vi "Process.vi"(8 "error in":errorcluster, 11 "Measurement.WavelengthSweeping":refnum<class "Measurement.WavelengthSweeping.lvclass">) -> (0 "error out":errorcluster, 3 "Measurement.WavelengthSweeping out":refnum<class "Measurement.WavelengthSweeping.lvclass">)   [LabVIEW 2017, in "Measurement.WavelengthSweeping.lvclass"]
doc: "---------------------------------------------------------------\nJKI State Machine Objects™\nhttp://jki.net/state-machine-objects/\nCopyright (C) 2005-2015, JKI <info@jki.net>\nALL RIGHTS RESERVEDJKI State Machine Objects (SMO) 1.0.0.5\nJKI - JKI\nCopyright (c) 2016, JKI"
uses:
  Measurement.WavelengthSweeping.lvclass
  D:/Program Files (x86)/National Instruments/LabVIEW 2017/vi.lib/JKI/JKI SMO/SMO/SMO.lvclass
  D:/upwork/Laser Measurement Tool/Laser/project/Subsystems/Measurement/Measurement.lvclass
  <vilib>/JKI/JKI SMO/SMO/Typedefs/Parent Call--Enum.ctl
  Measurement/Typedefs/Measurement.State--Enum.ctl
  OPA/Typedefs/PrivateEvents--OPA.SetShutterState.ctl
  Typedefs/Measurement.WavelengthSweeping.State--Enum.ctl
  Typedefs/Measurement.WavelengthSweeping.Measured--Data.ctl
  Measurement/Typedefs/PublicEvents--Measurement.Finished.ctl
  Measurement/Typedefs/PublicEvents--Measurement.Initialized.ctl
  <vilib>/Analysis/baseanly.llb/Mean (DBL).vi
  SMU/SMU.lvclass
  D:/upwork/Laser Measurement Tool/Laser/project/Subsystems/MeasuringDevice/MeasuringDevice.lvclass
  LIA/LIA.lvclass
  OPM/OPM.lvclass
  Measurement/Measurement.lvclass
  <vilib>/JKI/JKI SMO/SMO/SMO.lvclass
  OPA/OPA.lvclass
  MeasuringDevice/MeasuringDevice.lvclass
  <vilib>/Analysis/NI_AALBase.lvlib
panel:
  # "Measurement.WavelengthSweeping\nProcess.vi"
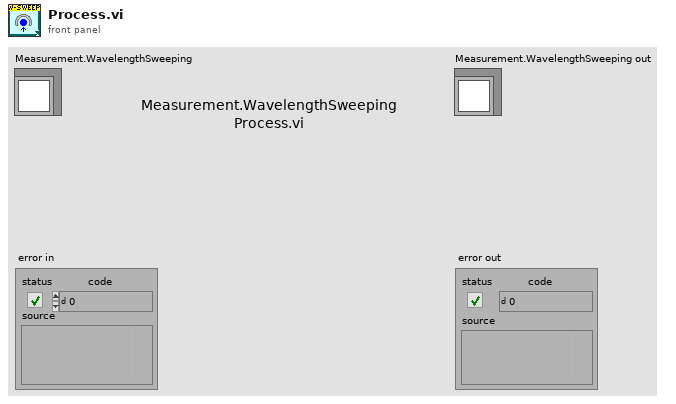
[diagram p1: front panel]
types:
  T1 = typedef "SMO.lvclass/Parent Call--Enum.ctl" = enum16{"Allows parent to run", "Does not request parent to run"}
  T2 = typedef "Measurement.lvclass/Measurement.State--Enum.ctl" = enum16{"Uninitialized", "Initialized", "Started", "Paused", "Stopped"}
  T3 = typedef "OPA.lvclass/PrivateEvents--OPA.SetShutterState.ctl" = bool
  T4 = typedef "Measurement.WavelengthSweeping.lvclass/Measurement.WavelengthSweeping.State--Enum.ctl" = enum16{"Stoppped", "Wait for Wavelength set", "Wait for Integration time", "Wait for Measurements", "Wait for Delay time"}
  T5 = enum32{"invalid app kind", "Development System", "Run Time System", "Student Edition", "Embedded LabVIEW", "Evaluation", "Custom"}
  T6 = enum32{"Invalid", "Standard", "Closed", "Hidden", "Minimized", "Maximized"}
  T7 = typedef "Measurement.lvclass/PublicEvents--Measurement.Finished.ctl" = bool
  T8 = typedef "Measurement.lvclass/PublicEvents--Measurement.Initialized.ctl" = bool
  T9 = typedef "Measurement.WavelengthSweeping.lvclass/Dependencies--Cluster.ctl" = cluster{"SMU":refnum<class "SMU.lvclass">, "LIA":refnum<class "LIA.lvclass">, "OPM":refnum<class "OPM.lvclass">, "OPA":refnum<class "OPA.lvclass">}
  T10 = typedef "Measurement.WavelengthSweeping.lvclass/Configuration--Cluster.ctl" = cluster{"Measurement.Type":T11, "Hardware":T12, "Measurement":T21}
  T11 = typedef "Measurement.lvclass/Measurement.Type--Enum.ctl" = enum16{"Free", "I/V Curve", "Wavelength sweeping", "Photocurrent mapping"}
  T12 = typedef "Measurement.WavelengthSweeping.lvclass/Configuration.Hardware--Cluster.ctl" = cluster{"SMU":T13, "LIA":T15, "OPM":T17, "OPA":T19}
  T13 = typedef "Measurement.lvclass/Configuration.SMU--Cluster.ctl" = cluster{"Enable":bool, "SMU Model":string, "Configuration":T14}
  T14 = typedef "SMU.lvclass/Configuration--Cluster.ctl" = cluster{"VISA Resource":string, "Channel":string}
  T15 = typedef "Measurement.lvclass/Configuration.LIA--Cluster.ctl" = cluster{"Enable":bool, "LIA Model":string, "Configuration":T16}
  T16 = typedef "LIA.lvclass/Configuration--Cluster.ctl" = cluster{"VISA Resource":string}
  T17 = typedef "Measurement.lvclass/Configuration.OPM--Cluster.ctl" = cluster{"Enable":bool, "OPM Model":string, "Configuration":T18}
  T18 = typedef "OPM.lvclass/Configuration--Cluster.ctl" = cluster{"VISA Resource":string}
  T19 = typedef "Measurement.lvclass/Configuration.OPA--Cluster.ctl" = cluster{"Enable":bool, "OPA Model":string, "Configuration":T20}
  T20 = typedef "OPA.lvclass/Configuration--Cluster.ctl" = cluster{"Serial Number":string}
  T21 = typedef "Measurement.WavelengthSweeping.lvclass/Configuration.Measurement--Cluster.ctl" = cluster{"SMU Voltage, V":dbl, "OPA Start wavelength, nm":dbl, "OPA Stop wavelength, nm":dbl, "OPA Scan resolution, nm":dbl, "OPA Number or points":u16, "Integration time, sec":dbl, "Delay time, ms":u16, "Accumulation":u16}
  T22 = cluster{"Core":cluster{"Current VI Reference":refnum<vi>, "Close Panel on Exit?":bool, "error":errorcluster}, "Self Reference":refnum<class "Measurement.WavelengthSweeping.lvclass">, "Dependencies":T9, "Configuration":T10, "Initialized":bool, "Meas State":T2, "W-Sweep State":T4, "Flags":cluster{"SMU Completed":bool, "LIA Completed":bool, "OPM Completed":bool, "OPA Wavelength":bool, "OPA Shutter State":bool}, "Next Step":string, "Wavelength, nm":dbl, "Start Time":timestamp, "SMU Measurement":dbl, "LIA Measurement":dbl, "OPM Measurement":dbl}
  T23 = cluster{"SMU Completed":bool, "LIA Completed":bool, "OPM Completed":bool, "OPA Wavelength":bool, "OPA Shutter State":bool}
  T24 = cluster{"Current VI Reference":refnum<vi>, "Close Panel on Exit?":bool, "error":errorcluster}
  T25 = typedef "Measurement.WavelengthSweeping.lvclass/Measurement.WavelengthSweeping.Measured--Data.ctl" = cluster{"Wavelength, nm":dbl, "Power, W":dbl, "Current, A":dbl, "Magnitude":dbl}
  T26 = typedef "SMO.lvclass/Protected Events.ctl" = cluster{"StopProcesses":refnum<user-event>, "AbortProcesses":refnum<user-event>, "Config Changed":refnum<user-event>, "Dependency":refnum<user-event>}
  T27 = cluster{"Event Registration Refnum":refnum<event-registration>, "Measurement Protected Events":refnum<event-registration>, "SMU Public Events":refnum<event-registration>, "LIA Public Events":refnum<event-registration>, "OPM Public Events":refnum<event-registration>, "OPA Public Events":refnum<event-registration>}
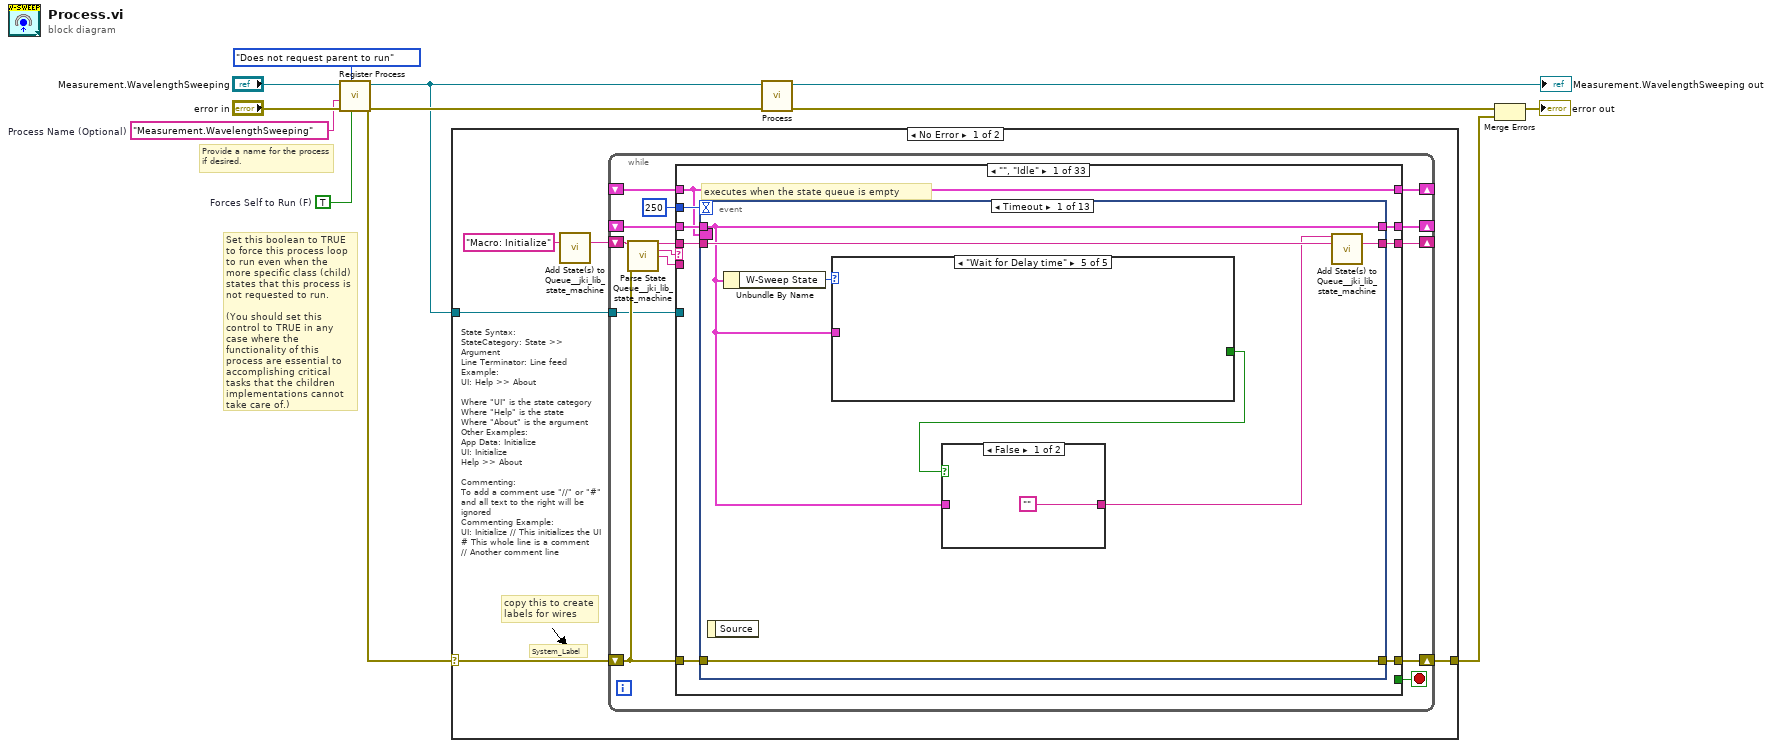
[diagram p0: block diagram]
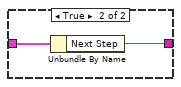
[diagram p2: hidden frame]
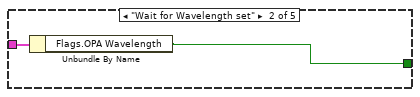
[diagram p4: hidden frame]
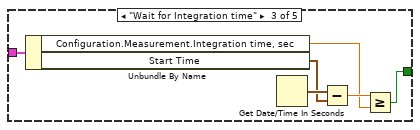
[diagram p5: hidden frame]
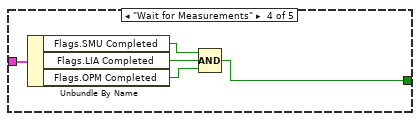
[diagram p6: hidden frame]
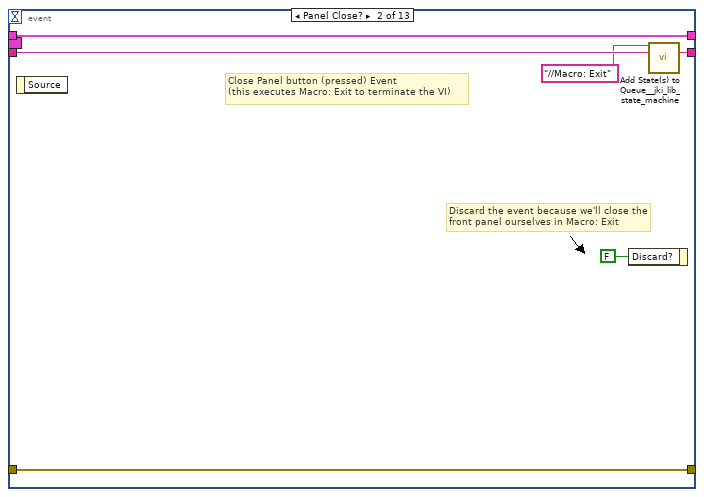
[diagram p7: hidden frame]
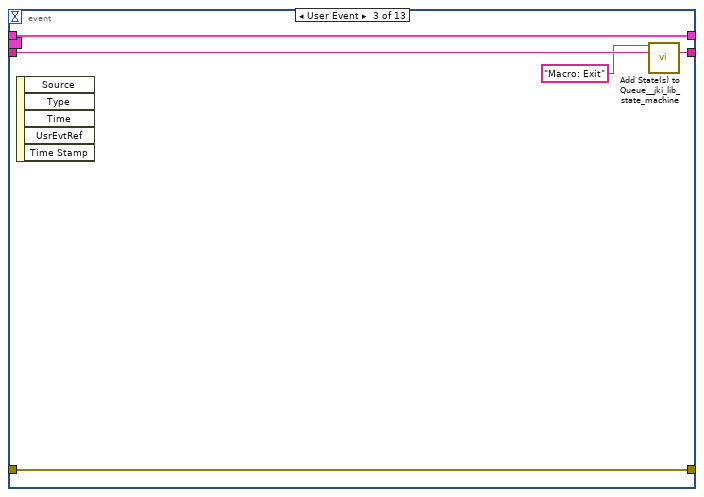
[diagram p8: hidden frame]
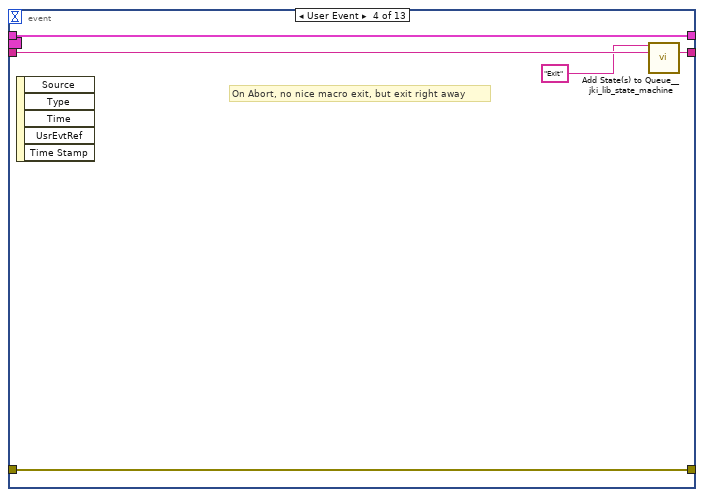
[diagram p9: hidden frame]
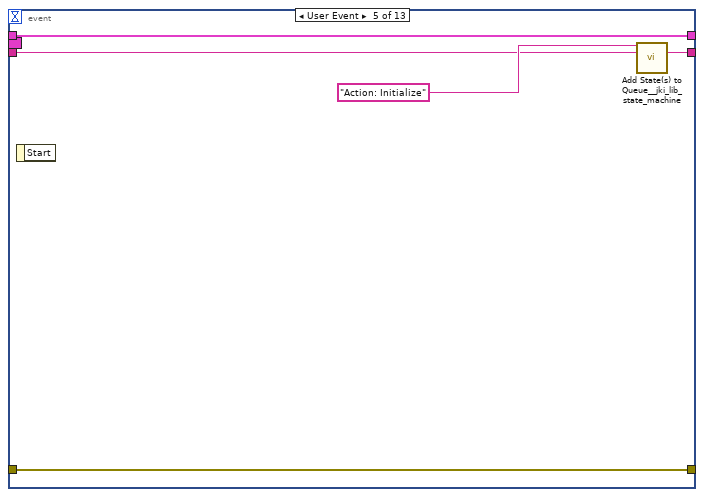
[diagram p10: hidden frame]
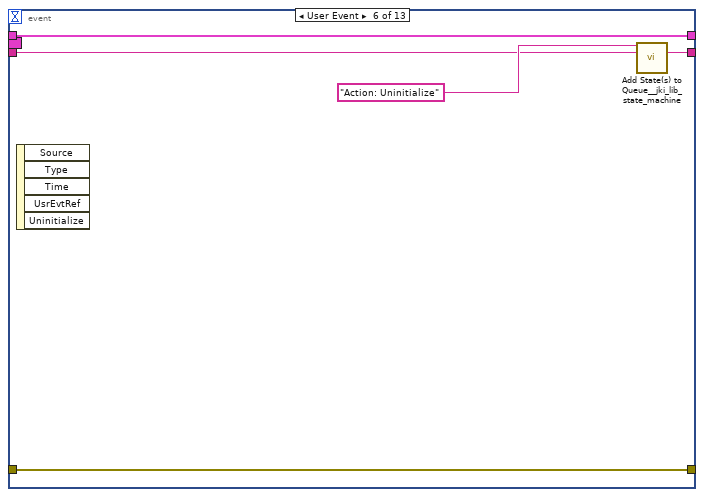
[diagram p11: hidden frame]
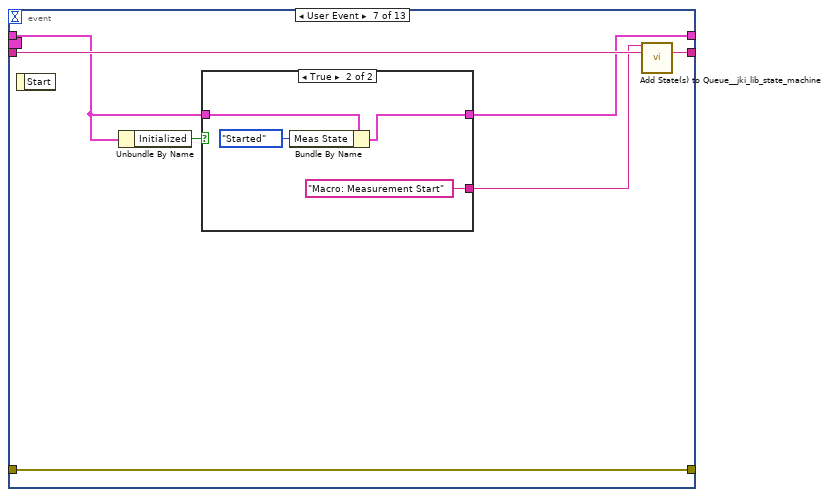
[diagram p12: hidden frame]
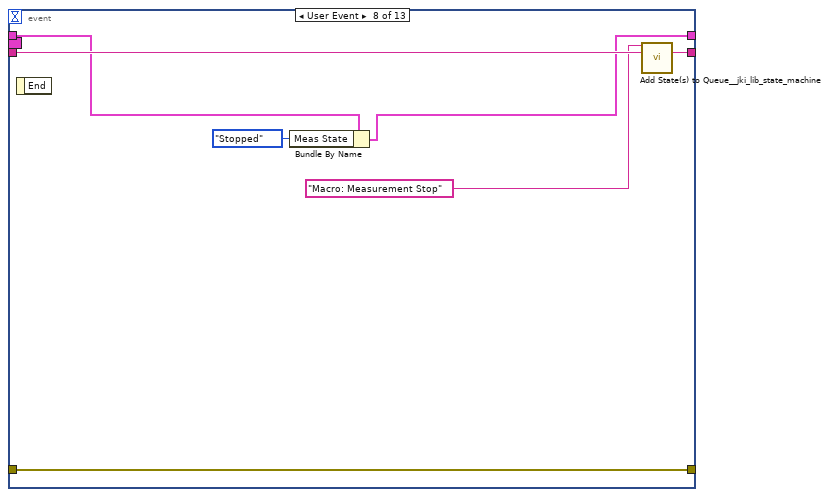
[diagram p14: hidden frame]
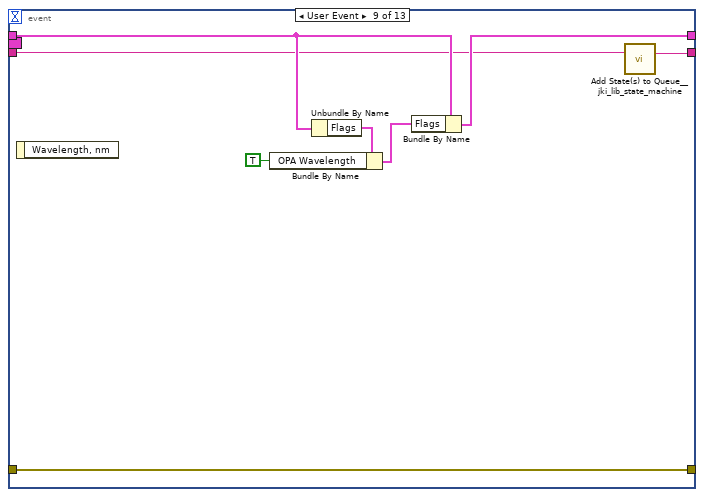
[diagram p15: hidden frame]
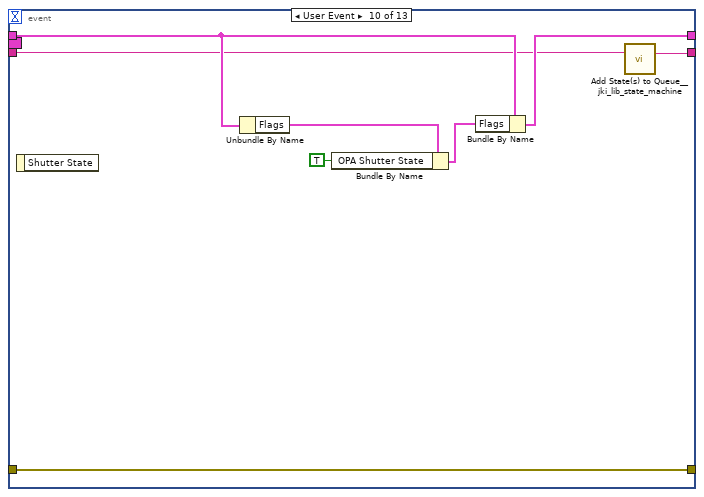
[diagram p16: hidden frame]
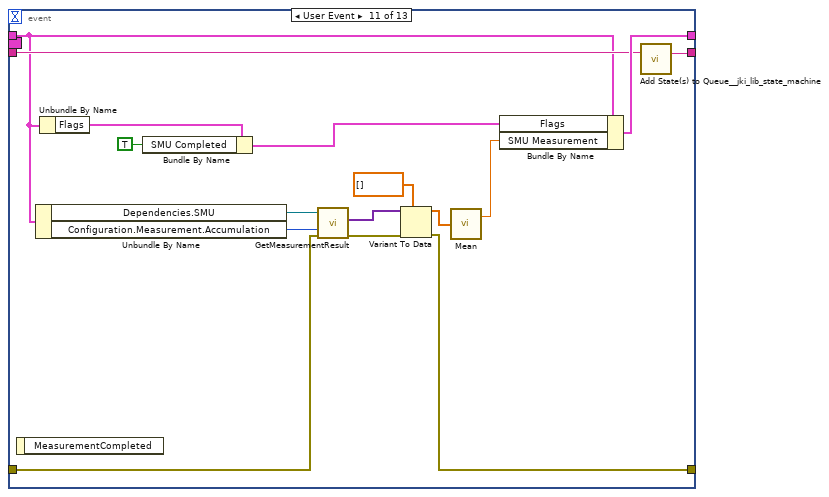
[diagram p17: hidden frame]
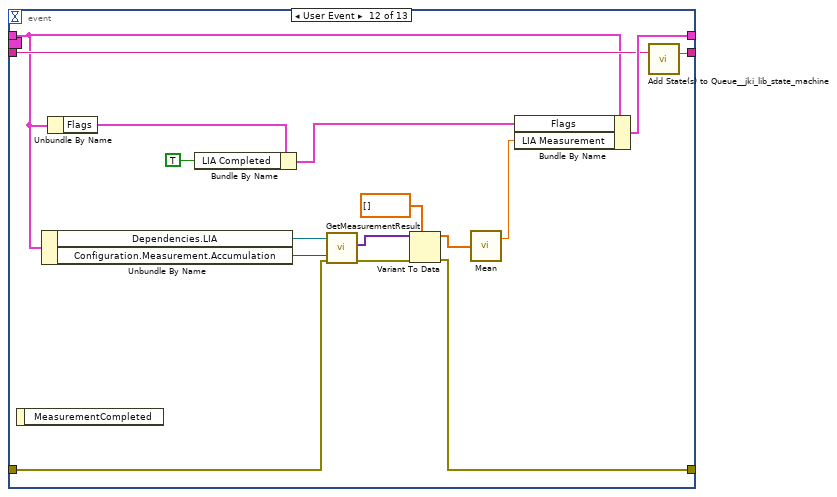
[diagram p18: hidden frame]
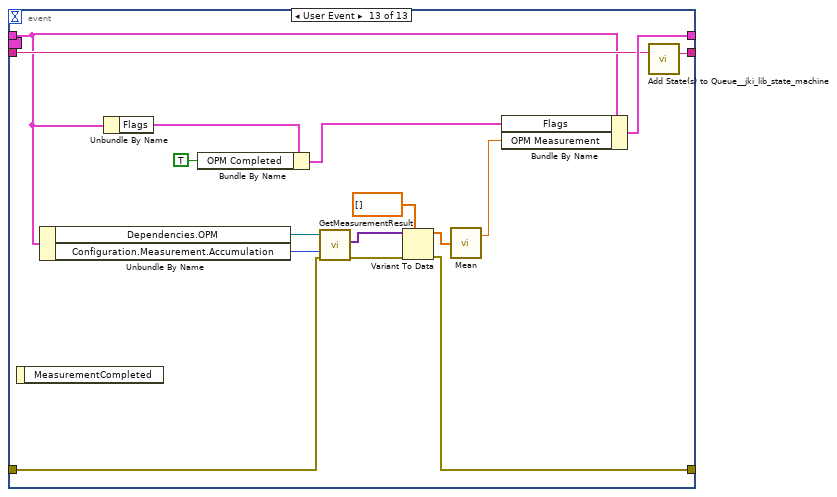
[diagram p19: hidden frame]
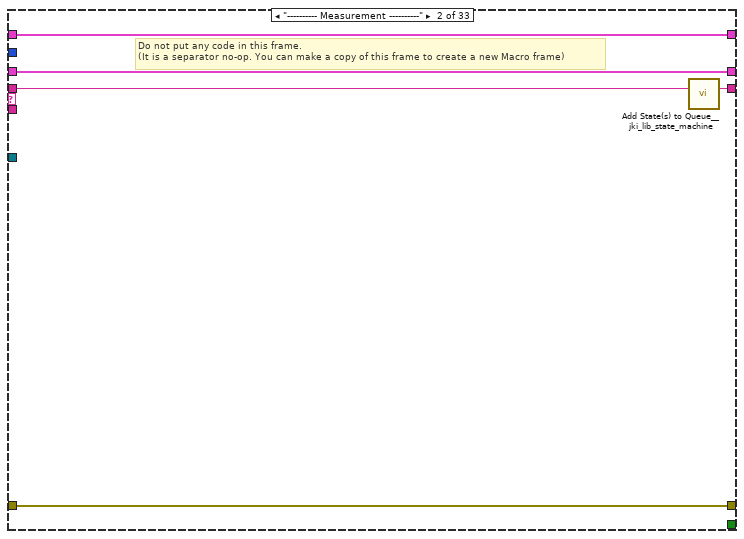
[diagram p20: hidden frame]
diagram:
  w2 = TRUE  # Forces Self to Run (F)
  w1 = "Measurement.WavelengthSweeping"  # Process Name (Optional)
  # "Provide a name for the process\nif desired."
  # "Set this boolean to TRUE to force this process loop to run even when the more specific class (child) states that this process is not requested to run.\n\n(You should set this control to TRUE in any case where the functionality of this process are essential to accomplishing critical tasks that the children implementations cannot take care of.)"
  n1 = call <vilib>:"Register Process.vi"("Forces Self to Run (F)"=w2, "Parent Call"=Parent_Call--Enum."Does not request parent to run", "error in (no error)"="error in", "Process Name (optional)"=w1, "SMO"="Measurement.WavelengthSweeping") -> ("error out"=w8:errorcluster, "SMO out"=w7:refnum<class "Measurement.WavelengthSweeping.lvclass">)  [unwired: 5 in]
  n2 = case shown="No Error" w8 {
    selector: w8 -> [w13 w662]
    tunnel: w7 -> [w14 _]
    tunnel: [w12 w662] -> w4
    frame No Error {
      # "State Syntax:\nStateCategory: State >> Argument\nLine Terminator: Line feed\nExample:\nUI: Help >> About\n\nWhere \"UI\" is the state category\nWhere \"Help\" is the state\nWhere \"About\" is the argument\nOther Examples:\nApp Data: Initialize\nUI: Initialize\nHelp >> About\n\nCommenting:\nTo add a comment use \"//\" or \"#\" and all text to the right will be ignored\nCommenting Example:\nUI: Initialize // This initializes the UI\n# This whole line is a comment\n// Another comment line"
      # "copy this to create labels for wires"
      # "System_Label"
      n3 = call <vilib>:"Add State(s) to Queue__jki_lib_state_machine.vi"("State(s) in (\"\")"="Macro: Initialize") -> ("States Out"=w16:string)  [unwired: 14 in]
      n4 = while {
        shift-right: [w23] -> _
        shift-left: _ -> [w22]
        shift-right: [w26] -> w12
        shift-left: w13 -> [w20]
        shift-right: [w25] -> _
        shift-left: w16 -> [w27]
        tunnel: w14 -> [w19]
        shift-right: [w18] -> _
        shift-left: _ -> [w17]
        stop <- w24 stop-if-true
        n5 = call <vilib>:"Parse State Queue__jki_lib_state_machine.vi"("State Queue"=w27, "Error In (no error)"=w20) -> ("Remaining States"=w29:string, "Current State"=w30:string, "Arguments"=w28:string)  [unwired: 11 in]
        n6 = case shown="\"\", \"Idle\"" w30 {
          selector: w30 -> [_ _ w176 w207 w258 w282 _ _ w363 _ _ _ _ _ _ _ _ _ _ _ _ _ _ _ _ _ _ _ _ _ _ _ _]
          tunnel: w29 -> [w38 w175 w183 w215 w264 w291 w348 w361 w367 w386 w401 w407 w412 w437 w444 w449 w454 w461 w477 w518 w523 w532 w546 w558 w571 w576 w587 w592 w617 w623 w628 w641 w661]
          tunnel: w28 -> [_ _ w181 w213 w261 w288 _ _ _ _ _ _ _ _ _ _ _ w455 w471 _ _ _ _ _ _ _ _ _ _ _ _ _ _]
          tunnel: w22 -> [w36 w172 w179 w211 w260 w284 w340 w358 w365 w377 w391 w403 w409 _ w439 w446 w452 w459 w473 w515 w520 w528 w537 w553 w563 w573 w584 w589 w596 w621 w626 w633 w652]
          tunnel: [w35 w173 w177 w209 w256 w285 w346 w359 w369 w383 w393 w402 w410 w425 w440 w447 w451 w456 w474 w507 w521 w530 w544 w556 w560 w574 w578 w590 w612 w619 w624 w629 w654] -> w26
          tunnel: w20 -> [w34 w173 w178 w210 w257 w286 w346 w359 w368 w383 w388 _ w410 w434 w441 w447 w451 w457 w475 w508 w521 w530 w544 w556 w561 w574 w579 w590 w597 w619 w624 w637 w657]
          tunnel: [w37 w174 w182 w214 w263 w290 w347 w360 w366 w385 w400 w406 w411 w436 w443 w448 w453 w460 w476 w517 w522 w531 w545 w557 w570 w575 w586 w591 w616 w622 w627 w640 w660] -> w25
          tunnel: [_ _ _ _ _ _ _ _ _ _ _ TRUE _ _ _ _ _ _ _ _ _ _ _ _ _ _ _ _ _ _ _ _ _] -> w24
          tunnel: [w33 w172 w179 w208 w259 w283 w338 w358 w365 w384 w390 w403 w409 w435 w439 w446 w452 w459 w473 w515 w520 w528 w537 w552 w564 w573 w584 w589 w596 w621 w626 w632 w651] -> w23
          tunnel: 250 ("Timeout") -> [w32 _ _ _ _ _ _ _ _ _ _ _ _ _ _ _ _ _ _ _ _ _ _ _ _ _ _ _ _ _ _ _ _]
          tunnel: w19 -> [_ _ _ _ _ _ _ _ _ _ _ _ _ w432 _ _ _ _ _ _ _ _ _ _ _ _ _ _ _ _ _ w638 w658]
          tunnel: [w31 w171 w180 w212 w262 w289 w345 w357 w362 w374 w399 w404 w408 w431 w438 w445 w450 w458 w470 w516 w519 w529 w538 w555 w569 w572 w585 w588 w611 w620 w625 w639 w659] -> w18
          tunnel: w17 -> [w31 w171 w180 w212 w262 w289 w345 w357 w362 w374 w399 w404 w408 w431 w438 w445 w450 w458 w470 w516 w519 w529 w538 w555 w569 w572 w585 w588 _ w620 w625 w639 w659]
          frame "", "Idle" {
            # "executes when the state queue is empty"
            n7 = event shown="[0] Timeout" {
              selector: w31 -> [_ _ _ _ _ _ _ _ _ _ _ _ _]
              dyn-events: _ -> [_ _ _ _ _ _ _ _ _ _ _ _ _]
              timeout: w32 -> [_ _ _ _ _ _ _ _ _ _ _ _ _]
              tunnel: w38 -> [w45 w67 w72 w77 w78 w83 w93 w105 w107 w115 w133 w149 w165]
              tunnel: [w44 w66 w71 w76 w80 w85 w94 w106 w108 w116 w134 w150 w166] -> w37
              tunnel: w36 -> [w40 w64 w69 w74 w81 w86 w89 w102 w113 w121 w132 w145 w161]
              tunnel: [w43 w65 w70 w75 w82 w87 w92 w104 w109 w117 w127 w143 w159] -> w35
              tunnel: w34 -> [w43 w65 w70 w75 w82 w87 w92 w104 w109 w117 w130 w144 w160]
              tunnel: [w40 w64 w69 w74 w81 w86 w88 w101 w114 w122 w138 w154 w170] -> w33
              event Timeout {
                n8 = event-data() -> ()  [unwired: 1 in, 1 out]
                n9 = Unbundle By Name(w40) -> ("W-Sweep State"=w42:T4)
                n10 = case shown="\"Wait for Delay time\"" w42 {
                  tunnel: w40 -> [_ w50 w52 w61 _]
                  tunnel: [_ w49 w51 w57 _] -> w41
                  frame "Stoppped", Default {
                  }
                  frame "Wait for Wavelength set" {
                    n11 = Unbundle By Name(w50) -> ("Flags.OPA Wavelength"=w49:bool)
                  }
                  frame "Wait for Integration time" {
                    n12 = Unbundle By Name(w52) -> ("Configuration.Measurement.Integration time, sec"=w53:dbl, "Start Time"=w55:timestamp)
                    n13 = Get Date/Time In Seconds() -> (seconds since 1Jan1904=w56:timestamp)
                    n14 = Subtract(x=w56, y=w55) -> (x-y=w54:dbl)
                    n15 = Greater Or Equal?(x=w54, y=w53) -> (x >= y?=w51:bool)
                  }
                  frame "Wait for Measurements" {
                    n16 = Unbundle By Name(w61) -> ("Flags.SMU Completed"=w60:bool, "Flags.LIA Completed"=w59:bool, "Flags.OPM Completed"=w58:bool)
                    n17 = Compound Arithmetic op=AND(w60, w59, w58) -> (w57:bool)
                  }
                  frame "Wait for Delay time" {
                  }
                }
                n18 = case shown="False" w41 {
                  tunnel: w40 -> [_ w48]
                  tunnel: ["" w47] -> w39
                  frame False {
                  }
                  frame True {
                    n19 = Unbundle By Name(w48) -> ("Next Step"=w47:string)
                  }
                }
                n20 = call <vilib>:"Add State(s) to Queue__jki_lib_state_machine.vi"("State(s) in Front (\"\")"=w39, "State(s) in (\"\")"=w45) -> ("States Out"=w44:string)  [unwired: 13 in]
              }
              event Panel Close? {
                # "Discard the event because we'll close the front panel ourselves in Macro: Exit"
                # "Close Panel button (pressed) Event\n(this executes Macro: Exit to terminate the VI)"
                n21 = event-data() -> ()  [unwired: 1 in, 1 out]
                n22 = event-data("Discard?"=FALSE) -> ()  [unwired: 1 in, 1 out]
                n23 = call <vilib>:"Add State(s) to Queue__jki_lib_state_machine.vi"("State(s) in Front (\"\")"="//Macro: Exit", "State(s) in (\"\")"=w67) -> ("States Out"=w66:string)  [unwired: 13 in]
              }
              event User Event {
                n24 = event-data() -> ()  [unwired: 1 in, 5 out]
                n25 = call <vilib>:"Add State(s) to Queue__jki_lib_state_machine.vi"("State(s) in Front (\"\")"="Macro: Exit", "State(s) in (\"\")"=w72) -> ("States Out"=w71:string)  [unwired: 13 in]
              }
              event User Event {
                # "On Abort, no nice macro exit, but exit right away"
                n26 = event-data() -> ()  [unwired: 1 in, 5 out]
                n27 = call <vilib>:"Add State(s) to Queue__jki_lib_state_machine.vi"("State(s) in Front (\"\")"="Exit", "State(s) in (\"\")"=w77) -> ("States Out"=w76:string)  [unwired: 13 in]
              }
              event User Event {
                n28 = event-data() -> ()  [unwired: 1 in, 1 out]
                n29 = call <vilib>:"Add State(s) to Queue__jki_lib_state_machine.vi"("State(s) in Front (\"\")"="Action: Initialize", "State(s) in (\"\")"=w78) -> ("States Out"=w80:string)  [unwired: 13 in]
              }
              event User Event {
                n30 = event-data() -> ()  [unwired: 1 in, 5 out]
                n31 = call <vilib>:"Add State(s) to Queue__jki_lib_state_machine.vi"("State(s) in Front (\"\")"="Action: Uninitialize", "State(s) in (\"\")"=w83) -> ("States Out"=w85:string)  [unwired: 13 in]
              }
              event User Event {
                n32 = event-data() -> ()  [unwired: 1 in, 1 out]
                n33 = Unbundle By Name(w89) -> ("Initialized"=w90:bool)
                n34 = case shown="True" w90 {
                  tunnel: [_ "Macro: Measurement Start"] -> w91
                  tunnel: w89 -> [w95 w98]
                  tunnel: [w95 w96] -> w88
                  frame False {
                  }
                  frame True {
                    n35 = Bundle By Name(cluster=w98, "Meas State"=Measurement.State--Enum."Started") -> (w96:T22)
                  }
                }
                n36 = call <vilib>:"Add State(s) to Queue__jki_lib_state_machine.vi"("State(s) in Front (\"\")"=w91, "State(s) in (\"\")"=w93) -> ("States Out"=w94:string)  [unwired: 13 in]
              }
              event User Event {
                n37 = event-data() -> ()  [unwired: 1 in, 1 out]
                n38 = Bundle By Name(cluster=w102, "Meas State"=Measurement.State--Enum."Stopped") -> (w101:T22)
                n39 = call <vilib>:"Add State(s) to Queue__jki_lib_state_machine.vi"("State(s) in Front (\"\")"="Macro: Measurement Stop", "State(s) in (\"\")"=w105) -> ("States Out"=w106:string)  [unwired: 13 in]
              }
              event User Event {
                n40 = event-data() -> ()  [unwired: 1 in, 1 out]
                n41 = Unbundle By Name(w113) -> ("Flags"=w112:T23)
                n42 = Bundle By Name(cluster=w112, "OPA Wavelength"=TRUE) -> (w111:T23)
                n43 = Bundle By Name(cluster=w113, "Flags"=w111) -> (w114:T22)
                n44 = call <vilib>:"Add State(s) to Queue__jki_lib_state_machine.vi"("State(s) in (\"\")"=w107) -> ("States Out"=w108:string)  [unwired: 14 in]
              }
              event User Event {
                n45 = event-data() -> ()  [unwired: 1 in, 1 out]
                n46 = Unbundle By Name(w121) -> ("Flags"=w120:T23)
                n47 = Bundle By Name(cluster=w120, "OPA Shutter State"=TRUE ("OPA Wavelength")) -> (w119:T23)
                n48 = Bundle By Name(cluster=w121, "Flags"=w119) -> (w122:T22)
                n49 = call <vilib>:"Add State(s) to Queue__jki_lib_state_machine.vi"("State(s) in (\"\")"=w115) -> ("States Out"=w116:string)  [unwired: 14 in]
              }
              event User Event {
                n50 = event-data() -> ()  [unwired: 1 in, 1 out]
                n51 = Unbundle By Name(w132) -> ("Dependencies.SMU"=w131:refnum<class "SMU.lvclass">, "Configuration.Measurement.Accumulation"=w123:u16)
                n52 = Unbundle By Name(w132) -> ("Flags"=w137:T23)
                n53 = Bundle By Name(cluster=w137, "SMU Completed"=TRUE ("OPA Wavelength")) -> (w136:T23)
                n54 = call "GetMeasurementResult.vi"("error in (no error)"=w130, "Count (1)"=w123, "MeasuringDevice in"=w131) -> ("error out"=w128:errorcluster, "Result"=w129:variant[])  [unwired: 6 in, 1 out]
                n55 = Variant To Data(error in=w128, type=dbl[] [], Variant=w129) -> (data=w125:dbl[], error out=w127:errorcluster)
                n56 = call-poly <vilib>:"Mean.vi"("X"=w125) -> ("mean"=w124:dbl)  [unwired: 1 out]
                n57 = Bundle By Name(cluster=w132, "Flags"=w136, "SMU Measurement"=w124) -> (w138:T22)
                n58 = call <vilib>:"Add State(s) to Queue__jki_lib_state_machine.vi"("State(s) in (\"\")"=w133) -> ("States Out"=w134:string)  [unwired: 14 in]
              }
              event User Event {
                n59 = event-data() -> ()  [unwired: 1 in, 1 out]
                n60 = Unbundle By Name(w145) -> ("Dependencies.LIA"=w148:refnum<class "LIA.lvclass">, "Configuration.Measurement.Accumulation"=w139:u16)
                n61 = Unbundle By Name(w145) -> ("Flags"=w153:T23)
                n62 = Bundle By Name(cluster=w153, "LIA Completed"=TRUE ("OPA Wavelength")) -> (w152:T23)
                n63 = call "GetMeasurementResult.vi"("error in (no error)"=w144, "Count (1)"=w139, "MeasuringDevice in"=w148) -> ("error out"=w146:errorcluster, "Result"=w147:variant[])  [unwired: 6 in, 1 out]
                n64 = Variant To Data(error in=w146, type=dbl[] [], Variant=w147) -> (data=w142:dbl[], error out=w143:errorcluster)
                n65 = call-poly <vilib>:"Mean.vi"("X"=w142) -> ("mean"=w140:dbl)  [unwired: 1 out]
                n66 = Bundle By Name(cluster=w145, "Flags"=w152, "LIA Measurement"=w140) -> (w154:T22)
                n67 = call <vilib>:"Add State(s) to Queue__jki_lib_state_machine.vi"("State(s) in (\"\")"=w149) -> ("States Out"=w150:string)  [unwired: 14 in]
              }
              event User Event {
                n68 = event-data() -> ()  [unwired: 1 in, 1 out]
                n69 = Unbundle By Name(w161) -> ("Dependencies.OPM"=w164:refnum<class "OPM.lvclass">, "Configuration.Measurement.Accumulation"=w155:u16)
                n70 = Unbundle By Name(w161) -> ("Flags"=w169:T23)
                n71 = Bundle By Name(cluster=w169, "OPM Completed"=TRUE ("OPA Wavelength")) -> (w168:T23)
                n72 = call "GetMeasurementResult.vi"("error in (no error)"=w160, "Count (1)"=w155, "MeasuringDevice in"=w164) -> ("error out"=w162:errorcluster, "Result"=w163:variant[])  [unwired: 6 in, 1 out]
                n73 = Variant To Data(error in=w162, type=dbl[] [], Variant=w163) -> (data=w157:dbl[], error out=w159:errorcluster)
                n74 = call-poly <vilib>:"Mean.vi"("X"=w157) -> ("mean"=w156:dbl)  [unwired: 1 out]
                n75 = Bundle By Name(cluster=w161, "Flags"=w168, "OPM Measurement"=w156) -> (w170:T22)
                n76 = call <vilib>:"Add State(s) to Queue__jki_lib_state_machine.vi"("State(s) in (\"\")"=w165) -> ("States Out"=w166:string)  [unwired: 14 in]
              }
            }
          }
          frame "---------- Measurement ----------" {
            # "Do not put any code in this frame.\n(It is a separator no-op. You can make a copy of this frame to create a new Macro frame)"
            n77 = call <vilib>:"Add State(s) to Queue__jki_lib_state_machine.vi"("State(s) in (\"\")"=w175) -> ("States Out"=w174:string)  [unwired: 14 in]
          }
          frame "Measurement: SMU" {
            n78 = case shown="\"Set Output Enable\"" w181 {
              selector: w181 -> [_ _ _ w200]
              tunnel: w179 -> [w188 w193 w196 _]
              tunnel: w178 -> [w185 w190 w195 w205]
              tunnel: [w184 w189 w194 w204] -> w177
              tunnel: w176 -> [_ _ _ w201]
              frame "Set Voltage" {
                n79 = Unbundle By Name(w188) -> ("Dependencies.SMU"=w187:refnum<class "SMU.lvclass">, "Configuration.Measurement.SMU Voltage, V"=w186:dbl)
                n80 = call "SetVoltage.vi"("error in (no error)"=w185, "Voltage, V"=w186, "SMU in"=w187) -> ("error out"=w184:errorcluster)  [unwired: 7 in, 1 out]
              }
              frame "Set Output Enable" {
                n81 = Unbundle By Name(w193) -> ("Dependencies.SMU"=w192:refnum<class "SMU.lvclass">)
                n82 = call "SetOutput.vi"("error in (no error)"=w190, "Output (False)"=TRUE, "SMU in"=w192) -> ("error out"=w189:errorcluster)  [unwired: 7 in, 1 out]
              }
              frame "Set Output Disable" {
                n83 = Unbundle By Name(w196) -> ("Dependencies.SMU"=w198:refnum<class "SMU.lvclass">)
                n84 = call "SetOutput.vi"("error in (no error)"=w195, "Output (False)"=FALSE, "SMU in"=w198) -> ("error out"=w194:errorcluster)  [unwired: 7 in, 1 out]
              }
              frame "Error", Default {
                w202 = "\r\n"
                n85 = Concatenate Strings("Nonexistent state caused" ("source"), w202, w201, w202, w200) -> (w199:string)
                n86 = call <vilib>:"Error Cluster From Error Code.vi"("error in (no error)"=w205, "error message (\"\")"=w199, "error code (0)"=-8000 ("code")) -> ("error out"=w204:errorcluster)  [unwired: 6 in]
              }
            }
            n87 = call <vilib>:"Add State(s) to Queue__jki_lib_state_machine.vi"("State(s) in (\"\")"=w183) -> ("States Out"=w182:string)  [unwired: 14 in]
          }
          frame "Measurement: OPA" {
            n88 = case shown="\"Set Wavelength\"" w213 {
              selector: w213 -> [_ _ _ w250]
              tunnel: w211 -> [w222 w229 w238 w247]
              tunnel: w210 -> [w219 w235 w244 w249]
              tunnel: [w218 w234 w243 w248] -> w209
              tunnel: [w223 w230 w239 w247] -> w208
              tunnel: w207 -> [_ _ _ w251]
              frame "Set Wavelength" {
                n89 = Unbundle By Name(w222) -> ("Dependencies.OPA"=w228:refnum<class "OPA.lvclass">, "Wavelength, nm"=w227:dbl)
                n90 = Unbundle By Name(w222) -> ("Dependencies.OPM"=w220:refnum<class "OPM.lvclass">, "Wavelength, nm"=w221:dbl)
                n91 = Unbundle By Name(w222) -> ("Flags"=w226:T23)
                n92 = Bundle By Name(cluster=w226, "OPA Wavelength"=FALSE) -> (w225:T23)
                n93 = call "SetWavelength.vi"("error in (no error)"=w219, "Wavelength"=w221, "OPM in"=w220) -> ("error out"=w216:errorcluster)  [unwired: 7 in, 1 out]
                n94 = call "SetWavelength.vi"("error in (no error)"=w219, "Wavelength, nm"=w227, "OPA in"=w228) -> ("error out"=w217:errorcluster)  [unwired: 7 in, 1 out]
                n95 = Bundle By Name(cluster=w222, "Flags"=w225) -> (w223:T22)
                n96 = Merge Errors(w216, w217) -> (w218:errorcluster)
              }
              frame "Set Shutter state Open" {
                n97 = Unbundle By Name(w229) -> ("Dependencies.OPA"=w237:refnum<class "OPA.lvclass">)
                n98 = Unbundle By Name(w229) -> ("Flags"=w233:T23)
                n99 = Bundle By Name(cluster=w233, "OPA Shutter State"=FALSE ("OPA Wavelength")) -> (w232:T23)
                n100 = call "SetShutterState.vi"("error in (no error)"=w235, "Shutter State"=T3 TRUE, "OPA"=w237) -> ("error out"=w234:errorcluster)  [unwired: 7 in, 1 out]
                n101 = Bundle By Name(cluster=w229, "Flags"=w232) -> (w230:T22)
              }
              frame "Set Shutter state Close" {
                n102 = Unbundle By Name(w238) -> ("Dependencies.OPA"=w246:refnum<class "OPA.lvclass">)
                n103 = Unbundle By Name(w238) -> ("Flags"=w242:T23)
                n104 = Bundle By Name(cluster=w242, "OPA Shutter State"=FALSE ("OPA Wavelength")) -> (w241:T23)
                n105 = call "SetShutterState.vi"("error in (no error)"=w244, "Shutter State"=T3 FALSE, "OPA"=w246) -> ("error out"=w243:errorcluster)  [unwired: 7 in, 1 out]
                n106 = Bundle By Name(cluster=w238, "Flags"=w241) -> (w239:T22)
              }
              frame "Error", Default {
                w253 = "\r\n"
                n107 = Concatenate Strings("Nonexistent state caused" ("source"), w253, w251, w253, w250) -> (w252:string)
                n108 = call <vilib>:"Error Cluster From Error Code.vi"("error in (no error)"=w249, "error message (\"\")"=w252, "error code (0)"=-8000 ("code")) -> ("error out"=w248:errorcluster)  [unwired: 6 in]
              }
            }
            n109 = call <vilib>:"Add State(s) to Queue__jki_lib_state_machine.vi"("State(s) in (\"\")"=w215) -> ("States Out"=w214:string)  [unwired: 14 in]
          }
          frame "Measurement: Pause" {
            n110 = case shown="\"Integration time\"" w261 {
              selector: w261 -> [_ _ w273]
              tunnel: w260 -> [w266 w272 w281]
              tunnel: [w266 w270 w281] -> w259
              tunnel: w258 -> [_ _ w274]
              tunnel: w257 -> [w265 w267 w276]
              tunnel: [w265 w267 w275] -> w256
              frame "Delay time" {
              }
              frame "Integration time" {
                n111 = Get Date/Time In Seconds() -> (seconds since 1Jan1904=w271:timestamp)
                n112 = Bundle By Name(cluster=w272, "Start Time"=w271, "W-Sweep State"=Measurement.WavelengthSweeping.State--Enum."Wait for Integration time", "Next Step"="Measurement: Measure >> All") -> (w270:T22)
              }
              frame "Error", Default {
                w278 = "\r\n"
                n113 = Concatenate Strings("Nonexistent state caused" ("source"), w278, w274, w278, w273) -> (w277:string)
                n114 = call <vilib>:"Error Cluster From Error Code.vi"("error in (no error)"=w276, "error message (\"\")"=w277, "error code (0)"=-8000 ("code")) -> ("error out"=w275:errorcluster)  [unwired: 6 in]
              }
            }
            n115 = call <vilib>:"Add State(s) to Queue__jki_lib_state_machine.vi"("State(s) in (\"\")"=w264) -> ("States Out"=w263:string)  [unwired: 14 in]
          }
          frame "Measurement: Measure" {
            n116 = case shown="\"All\"" w288 {
              selector: w288 -> [_ _ _ _ w331]
              tunnel: ["Measurement: Measure >> SMU\nMeasurement: Measure >> LIA\nMeasurement: Measure >> OPM" ("Next Step") _ _ _ _] -> w287
              tunnel: w284 -> [_ w307 w317 w327 _]
              tunnel: w286 -> [w296 w305 w315 w325 w330]
              tunnel: [w296 w304 w314 w324 w329] -> w285
              tunnel: w284 -> [w295 w300 w310 w320 w328]
              tunnel: [w294 w299 w309 w319 w328] -> w283
              tunnel: w282 -> [_ _ _ _ w332]
              frame "All" {
                n117 = Bundle By Name(cluster=w295, "W-Sweep State"=Measurement.WavelengthSweeping.State--Enum."Wait for Measurements", "Next Step"="UI: Send to UI\nMeasurement: Next Step") -> (w294:T22)
              }
              frame "SMU" {
                n118 = Unbundle By Name(w307) -> ("Dependencies.SMU"=w306:refnum<class "SMU.lvclass">, "Configuration.Measurement.Accumulation"=w298:u16)
                n119 = Unbundle By Name(w300) -> ("Flags"=w303:T23)
                n120 = call "Measure.vi"("error in (no error)"=w305, "Count (1)"=w298, "MeasuringDevice"=w306) -> ("error out"=w304:errorcluster)  [unwired: 6 in, 2 out]
                n121 = Bundle By Name(cluster=w303, "SMU Completed"=FALSE) -> (w301:T23)
                n122 = Bundle By Name(cluster=w300, "Flags"=w301) -> (w299:T22)
              }
              frame "LIA" {
                n123 = Unbundle By Name(w317) -> ("Dependencies.LIA"=w316:refnum<class "LIA.lvclass">, "Configuration.Measurement.Accumulation"=w308:u16)
                n124 = Unbundle By Name(w310) -> ("Flags"=w313:T23)
                n125 = call "Measure.vi"("error in (no error)"=w315, "Count (1)"=w308, "MeasuringDevice"=w316) -> ("error out"=w314:errorcluster)  [unwired: 6 in, 2 out]
                n126 = Bundle By Name(cluster=w313, "LIA Completed"=FALSE ("SMU Completed")) -> (w311:T23)
                n127 = Bundle By Name(cluster=w310, "Flags"=w311) -> (w309:T22)
              }
              frame "OPM" {
                n128 = Unbundle By Name(w327) -> ("Dependencies.OPM"=w326:refnum<class "OPM.lvclass">, "Configuration.Measurement.Accumulation"=w318:u16)
                n129 = Unbundle By Name(w320) -> ("Flags"=w323:T23)
                n130 = call "Measure.vi"("error in (no error)"=w325, "Count (1)"=w318, "MeasuringDevice"=w326) -> ("error out"=w324:errorcluster)  [unwired: 6 in, 2 out]
                n131 = Bundle By Name(cluster=w323, "OPM Completed"=FALSE ("SMU Completed")) -> (w321:T23)
                n132 = Bundle By Name(cluster=w320, "Flags"=w321) -> (w319:T22)
              }
              frame "Error", Default {
                w334 = "\r\n"
                n133 = Concatenate Strings("Nonexistent state caused" ("source"), w334, w332, w334, w331) -> (w333:string)
                n134 = call <vilib>:"Error Cluster From Error Code.vi"("error in (no error)"=w330, "error message (\"\")"=w333, "error code (0)"=-8000 ("code")) -> ("error out"=w329:errorcluster)  [unwired: 6 in]
              }
            }
            n135 = call <vilib>:"Add State(s) to Queue__jki_lib_state_machine.vi"("State(s) in Front (\"\")"=w287, "State(s) in (\"\")"=w291) -> ("States Out"=w290:string)  [unwired: 13 in]
          }
          frame "Measurement: Next Step" {
            n136 = Unbundle By Name(w340) -> ("Wavelength, nm"=w344:dbl, "Configuration.Measurement.OPA Scan resolution, nm"=w343:dbl, "Configuration.Measurement.OPA Stop wavelength, nm"=w342:dbl)
            n137 = Add(x=w344, y=w343) -> (x+y=w339:dbl)
            n138 = Less Or Equal?(x=w339, y=w342) -> (x <= y?=w341:bool)
            n139 = case shown="True" w341 {
              tunnel: w340 -> [w350 w356]
              tunnel: w339 -> [_ w355]
              tunnel: [w350 w354] -> w338
              tunnel: ["Macro: Measurement Stop" "Measurement: OPA >> Set Shutter state Close\nMeasurement: OPA >> Set Wavelength"] -> w337
              frame False {
                # "Stop measurement"
              }
              frame True {
                # "3. Do next"
                # "2. Wait for"
                # "1. Do now"
                # "Go to next wavelength"
                n140 = Bundle By Name(cluster=w356, "Wavelength, nm"=w355, "W-Sweep State"=Measurement.WavelengthSweeping.State--Enum."Wait for Wavelength set", "Next Step"="Measurement: OPA >> Set Shutter state Open\nMeasurement: Pause >>  Integration time") -> (w354:T22)
              }
            }
            n141 = call <vilib>:"Add State(s) to Queue__jki_lib_state_machine.vi"("State(s) in Front (\"\")"=w337, "State(s) in (\"\")"=w348) -> ("States Out"=w347:string)  [unwired: 13 in]
          }
          frame "---------- Core ----------" {
            # "Do not put any code in this frame.\n(it is a separator no-op)"
            n142 = call <vilib>:"Add State(s) to Queue__jki_lib_state_machine.vi"("State(s) in (\"\")"=w361) -> ("States Out"=w360:string)  [unwired: 14 in]
          }
          frame Default {
            w372 = 42 items=["No error", "Argument error", "Memory is full", "Out of zone", "End of file", "File already open", "Generic file I/O error", "File not found", "File permission error", "Disk is full", "Duplicate path", "Too many files open", "System feature not enabled", "Resource file not found", "Cannot add resource", "Resource not found", "Image not found", "Image memory error", "Pen does not exist", "Config type invalid", "Config token not found", "Config parse error", "Config memory error", "Bad external code format", "Bad external code offset", "External code not present", "Null window", "Destroy window error", "Null menu", "Print aborted", "Bad print record", "Print driver error", "Windows error during printing", "Memory error during printing", "Print dialog error", "Generic print error", "Invalid device refnum", "Device not found", "Device parameter error", "Device unit error", "Cannot open device", "Device call aborted", "Generic error", "Cancelled by user", "Object ID too low", "Object ID too high", "Object not in heap", "Unknown heap", "Unknown object (invalid DefProc)", "Unknown object (DefProc not in table)", "Message out of range", "Invalid (null) method", "Unknown message", "Manager call not supported", "Bad address", "Network operation in progress", "Network operation timed out", "Connection is busy", "Network attribute not supported", "Network error", "Address in use", "System out of memory", "Connection aborted", "Connection refused", "Not connected", "Already connected", "Connection closed", "Initialization error (interapplication manager)", "Bad occurrence", "Wait on unbound occurrence handler", "Occurrence queue overflow", "Datalog type conflict", "Unused", "Unrecognized type (interapplication manager)", "Memory corrupt", "Failed to make temporary DLL", "Old CIN version", "Drag socket not found", "Failed to load drop-object", "Failed to register OLE object", "Failed to release OLE object", "Format specifier type mismatch", "Unknown format specifier", "Too few format specifiers", "Too many format specifiers", "Scan failed", "Newer CIN version", "Error converting to variant", "Runtime menu error", "Password tampered", "Variant attribute not found", "Incompatible variant data type", "Event data is not available", "Event Store is not present", "Occurrence is not found", "Event Queue is not created", "Event info is not available", "Refnum passed is NULL", "Error retrieving Class GUID", "Error retrieving CoClass GUID", "Error retrieving TypeLib GUID.", "Bad built application magic bytes.", "Specific driver is different from the specific driver associated with the Logical Name.", "There is no session opened to the class driver.", "Max Error", "MAX - Error with config objects", "MAX - Error loading configuration", "MAX - Group not supported"]
            # "Current State"
            # "Do not delete, rename, or modify this frame.\n(this is used to capture unhandled states and typos)"
            # "Handle mistyped state name (developer tool)"
            n143 = Format Into String(format string="Software Exception: Unhandled State \"%s\"." ("message"), error in=w368, w363) -> (resulting string=w371:string, error out=w370:errorcluster)  [unwired: 1 in]
            n144 = call <vilib>:"Error Cluster From Error Code.vi"("show call chain? (False)"=TRUE, "error in (no error)"=w370, "error message (\"\")"=w371, "error code (0)"=w372) -> ("error out"=w369:errorcluster)  [unwired: 5 in]
            n145 = call <vilib>:"Add State(s) to Queue__jki_lib_state_machine.vi"("State(s) in (\"\")"=w367) -> ("States Out"=w366:string)  [unwired: 14 in]
          }
          frame "Initialize Core Data" {
            # "Do not delete, rename, or modify this frame.\n(this is used to determine panel behavior on exit)"
            # "originally closed?"
            # "exe?"
            # "If panel starts closed or is an EXE, then close it when we exit"
            n146 = property class="VI"() -> ("Front Panel.Open"=w382:bool)  [unwired: 2 in, 2 out]
            n147 = property class="App"() -> ("App.Kind"=w381:T5)  [unwired: 2 in, 2 out]
            n148 = control-ref of="Current VI Reference"() -> (w375:refnum<vi>)
            n149 = Not(x=w382) -> (.not. x?=w379:bool)
            n150 = Equal?(x=w381, y=T5."Run Time System" ("Application:Kind")) -> (x = y?=w378:bool)
            n151 = Or(x=w379, y=w378) -> (x .or. y?=w376:bool)
            n152 = Bundle By Name(cluster=w377, "Core.Current VI Reference"=w375, "Core.Close Panel on Exit?"=w376) -> (w384:T22)
            n153 = call <vilib>:"Add State(s) to Queue__jki_lib_state_machine.vi"("State(s) in (\"\")"=w386) -> ("States Out"=w385:string)  [unwired: 14 in]
          }
          frame "Error Handler" {
            w393 = errorcluster {"status"=FALSE, "code"=0, "source"=""}  # No error
            # "Overwrite this method to handle errors and pass to parent if not handled. Parent will fire a public event if the error is not handled up the chain of classes."
            # "Handle any errors here.\nYou can also output any states to clean-up after errors occur"
            n154 = Unbundle By Name(w391) -> ("Self Reference"=w398:refnum<class "Measurement.WavelengthSweeping.lvclass">)
            n155 = call <vilib>:"Simple Error Handler.vi"("error in (no error)"=w388) -> ("error out"=w387:errorcluster)  [unwired: 4 in, 4 out]
            n156 = call-dynamic "Handle Error.vi"("Stop on Unhandled Error (T)"=TRUE, "error in"=w387, "SMO"=w398) -> ("handling error"=w394:errorcluster, "Unhandled error"=w392:errorcluster)  [unwired: 6 in, 1 out]
            n157 = Bundle By Name(cluster=w391, "Core.error"=w392) -> (w390:T22)
            n158 = Select(t="Exit", s=w394, f="") -> (s? t:f=w395:string)
            n159 = call <vilib>:"Add State(s) to Queue__jki_lib_state_machine.vi"("State(s) in Front (\"\")"=w395, "State(s) in (\"\")"=w401) -> ("States Out"=w400:string)  [unwired: 13 in]
          }
          frame "Exit" {
            # "Do not put any code in this frame.\n(No errors that occur here will be handled.)"
            n160 = Unbundle By Name(w403) -> ("Core.error"=w402:errorcluster)
            n161 = call <vilib>:"Add State(s) to Queue__jki_lib_state_machine.vi"("State(s) in (\"\")"=w407) -> ("States Out"=w406:string)  [unwired: 14 in]
          }
          frame "---------- Data ----------" {
            # "Do not put any code in this frame.\n(It is a separator no-op. You can make a copy of this frame to create a new Data frame)"
            n162 = call <vilib>:"Add State(s) to Queue__jki_lib_state_machine.vi"("State(s) in (\"\")"=w412) -> ("States Out"=w411:string)  [unwired: 14 in]
          }
          frame "Data: Initialize" {
            w413 = 0.0  # OPM Measurement
            w414 = 0.0  # LIA Measurement
            w415 = 0.0  # SMU Measurement
            w416 = timestamp(0 s since 1904-01-01)  # Start Time
            w417 = 0.0  # Wavelength, nm
            w418 = ""  # Next Step
            w419 = T23 {"SMU Completed"=FALSE, "LIA Completed"=FALSE, "OPM Completed"=FALSE, "OPA Wavelength"=FALSE, "OPA Shutter State"=FALSE}  # Flags
            w420 = Measurement.WavelengthSweeping.State--Enum."Stoppped"  # W-Sweep State
            w421 = FALSE  # Initialized
            w422 = Measurement.State--Enum."Uninitialized"  # Meas State
            w430 = T24 {"Current VI Reference"=refnum, "Close Panel on Exit?"=FALSE, "error"={"status"=FALSE, "code"=0, "source"=""}}  # Core
            w433 = refnum<class "Measurement.WavelengthSweeping.lvclass"> refnum  # Self Reference
            # "do not delete - used by framework"
            # "Data names and types of shift register data are defined by this bundle."
            # "Initialize the shift-register data, here.\n(data names are defined by what you wire into the bundle function)"
            n163 = Variant To Data(error in=w434, type=w433, Variant=w432) -> (data=w429:refnum<class "Measurement.WavelengthSweeping.lvclass">, error out=w428:errorcluster)
            n164 = call "Measurement.WavelengthSweeping.GetStaticDependencies.vi"("error in (no error)"=w428, "Measurement.WavelengthSweeping in"=w429) -> ("error out"=w426:errorcluster, "Dependencies"=w424:T9, "Measurement.WavelengthSweeping out"=w427:refnum<class "Measurement.WavelengthSweeping.lvclass">)  [unwired: 7 in]
            n165 = call "Measurement.WavelengthSweeping.GetConfiguration.vi"("error in (no error)"=w426, "Measurement.WavelengthSweeping"=w427) -> ("error out"=w425:errorcluster, "Configuration"=w423:T10)  [unwired: 7 in, 1 out]
            n166 = Bundle("Core"=w430, "Self Reference"=w429, "Dependencies"=w424, "Configuration"=w423, "Initialized"=w421, "Meas State"=w422, "W-Sweep State"=w420, "Flags"=w419, "Next Step"=w418, "Wavelength, nm"=w417, "Start Time"=w416, "SMU Measurement"=w415, "LIA Measurement"=w414, "OPM Measurement"=w413) -> (w435:T22)  [unwired: 1 in]
            n167 = call <vilib>:"Add State(s) to Queue__jki_lib_state_machine.vi"("State(s) in (\"\")"=w437) -> ("States Out"=w436:string)  [unwired: 14 in]
          }
          frame "Data: Cleanup" {
            # "Cleanup any data and references, here.\n(this is called automatically, by the Macro: Exit)"
            n168 = Unbundle By Name(w439) -> ("Core.Current VI Reference"=w442:refnum<vi>)
            n169 = Close Reference(reference=w442, error in (no error)=w441) -> (error out=w440:errorcluster)
            n170 = call <vilib>:"Add State(s) to Queue__jki_lib_state_machine.vi"("State(s) in (\"\")"=w444) -> ("States Out"=w443:string)  [unwired: 14 in]
          }
          frame "---------- UI ----------" {
            # "Do not put any code in this frame.\n(It is a separator no-op. You can make a copy of this frame to create a new UI frame)"
            n171 = call <vilib>:"Add State(s) to Queue__jki_lib_state_machine.vi"("State(s) in (\"\")"=w449) -> ("States Out"=w448:string)  [unwired: 14 in]
          }
          frame "UI: Initialize" {
            # "Initialize the User Interface, here.\n(this is called automatically, by the Macro: Init)"
            n172 = call <vilib>:"Add State(s) to Queue__jki_lib_state_machine.vi"("State(s) in (\"\")"=w454) -> ("States Out"=w453:string)  [unwired: 14 in]
          }
          frame "UI: Cursor Set" {
            # "Argument"
            # "Initialize the User Interface, here.\n(this is called automatically, by the Macro: Init)"
            n173 = disable-structure shown="Default" {
              disable-tunnel: w457 -> [w462 w465]
              disable-tunnel: [w462 w464] -> w456
              disable-tunnel: w455 -> [_ w463]
              frame condition #0 {
              }
              frame condition #1 (active) {
                n174 = case shown="\"Busy\"" w463 {
                  tunnel: w465 -> [w467 w469]
                  tunnel: [w466 w468] -> w464
                  frame "Idle", Default {
                    n175 = call <vilib>:"Unset Busy.vi"("error in (no error)"=w467) -> ("error out"=w466:errorcluster)  [unwired: 10 in]
                  }
                  frame "Busy" {
                    n176 = call <vilib>:"Set Busy.vi"("error in (no error)"=w469) -> ("error out"=w468:errorcluster)  [unwired: 9 in, 1 out]
                  }
                }
              }
            }
            n177 = call <vilib>:"Add State(s) to Queue__jki_lib_state_machine.vi"("State(s) in (\"\")"=w461) -> ("States Out"=w460:string)  [unwired: 14 in]
          }
          frame "UI: Front Panel State" {
            # "Argument"
            # "Set Front Panel Open or Closed\n(Usage: \"UI: Front Panel State >> Open|Close\")"
            n178 = Unbundle By Name(w473) -> ("Core.Current VI Reference"=w472:refnum<vi>)
            n179 = disable-structure shown="Default" {
              disable-tunnel: w475 -> [w481 w504]
              disable-tunnel: [w480 w504] -> w474
              disable-tunnel: w472 -> [w479 _]
              disable-tunnel: w471 -> [w478 _]
              frame condition #0 (active) {
                n180 = case shown="\"Open\", Default" w478 {
                  tunnel: w481 -> [w485 w498]
                  tunnel: [w487 w499] -> w480
                  tunnel: w479 -> [w486 w496]
                  frame "Open", Default {
                    n181 = property class="VI"(reference=w486, error in=w485) -> (reference out=w483:refnum<vi>, error out=w484:errorcluster, "FP.State"=w482:T6)
                    n182 = case shown="\"Closed\"" w482 {
                      tunnel: [w490 w493] -> w487
                      tunnel: w484 -> [w489 w493]
                      tunnel: w483 -> [w488 _]
                      frame "Closed" {
                        n183 = invoke class="VI" method="FP.Open"(reference=w488, error in=w489, "Activate"=TRUE, "State"=T6."Standard") -> (error out=w490:errorcluster)  [unwired: 1 in, 4 out]
                      }
                      frame Default {
                      }
                    }
                  }
                  frame "Close" {
                    n184 = property class="VI"(reference=w496, error in=w498) -> (reference out=w495:refnum<vi>, error out=w497:errorcluster, "FP.State"=w494:T6)
                    n185 = case shown="Default" w494 {
                      tunnel: [w500 w503] -> w499
                      tunnel: w497 -> [w500 w502]
                      tunnel: w495 -> [_ w501]
                      frame "Invalid", "Closed" {
                      }
                      frame Default {
                        n186 = invoke class="VI" method="FP.Close"(reference=w501, error in=w502) -> (error out=w503:errorcluster)  [unwired: 1 in, 2 out]
                      }
                    }
                  }
                }
              }
              frame condition #1 {
              }
            }
            n187 = call <vilib>:"Add State(s) to Queue__jki_lib_state_machine.vi"("State(s) in (\"\")"=w477) -> ("States Out"=w476:string)  [unwired: 14 in]
          }
          frame "UI: Send to UI" {
            w506 = T25 {"Wavelength, nm"=0.0, "Power, W"=0.0, "Current, A"=0.0, "Magnitude"=0.0}  # Measurement.WavelengthSweeping.Measured
            n188 = Unbundle By Name(w515) -> ("Self Reference"=w514:refnum<class "Measurement.WavelengthSweeping.lvclass">, "Wavelength, nm"=w513:dbl, "SMU Measurement"=w511:dbl, "LIA Measurement"=w510:dbl, "OPM Measurement"=w512:dbl)
            n189 = Bundle By Name(cluster=w506, "Wavelength, nm"=w513, "Power, W"=w512, "Current, A"=w511, "Magnitude"=w510) -> (w509:T25)
            n190 = To Variant(anything=w509) -> (Variant=w505:variant)
            n191 = call "Measurement.OnMeasured.vi"("error in (no error)"=w508, "Payload"=w505, "Measurement in"=w514) -> ("error out"=w507:errorcluster)  [unwired: 7 in, 1 out]
            n192 = call <vilib>:"Add State(s) to Queue__jki_lib_state_machine.vi"("State(s) in (\"\")"=w518) -> ("States Out"=w517:string)  [unwired: 14 in]
          }
          frame "---------- Macro ----------" {
            # "Do not put any code in this frame.\n(It is a separator no-op. You can make a copy of this frame to create a new Macro frame)"
            n193 = call <vilib>:"Add State(s) to Queue__jki_lib_state_machine.vi"("State(s) in (\"\")"=w523) -> ("States Out"=w522:string)  [unwired: 14 in]
          }
          frame "Macro: Initialize" {
            w526 = "UI: Initialize\n//UI: Front Panel State >> Open"  # UI: Initialize //UI: Front Panel State >> Open
            # "Initialization Macro\n(This is called once, when the VI starts)"
            n194 = call <vilib>:"Add State(s) to Queue__jki_lib_state_machine.vi"("State(s) in Front (\"\")"="Data: Initialize\nInitialize Core Data\nEvents: Register", "State(s) in (\"\")"="Process: Sync", "State(s) at Back (\"\")"=w526) -> ("States Out"=w525:string)  [unwired: 12 in]
            n195 = call <vilib>:"Add State(s) to Queue__jki_lib_state_machine.vi"("State(s) in Front (\"\")"=w525, "State(s) in (\"\")"=w532) -> ("States Out"=w531:string)  [unwired: 13 in]
          }
          frame "Macro: Exit" {
            # "Exit Macro\n(This is called once, when the VI exits)"
            n196 = Unbundle By Name(w537) -> ("Core.Close Panel on Exit?"=w543:bool)
            n197 = Select(t="UI: Front Panel State >> Close", s=w543, f="") -> (s? t:f=w540:string)
            n198 = call <vilib>:"Add State(s) to Queue__jki_lib_state_machine.vi"("State(s) in Front (\"\")"="Data: Cleanup\nEvents: Unregister", "State(s) in (\"\")"="Process: Sync", "State(s) at Back (\"\")"="Exit") -> ("States Out"=w534:string)  [unwired: 12 in]
            n199 = call <vilib>:"Add State(s) to Queue__jki_lib_state_machine.vi"("State(s) in (\"\")"=w540, "State(s) at Back (\"\")"=w534) -> ("States Out"=w539:string)  [unwired: 13 in]
            n200 = call <vilib>:"Add State(s) to Queue__jki_lib_state_machine.vi"("State(s) in Front (\"\")"=w539, "State(s) in (\"\")"=w546) -> ("States Out"=w545:string)  [unwired: 13 in]
          }
          frame "Macro: Measurement Start" {
            n201 = Unbundle By Name(w553) -> ("Configuration.Measurement.OPA Start wavelength, nm"=w554:dbl)
            n202 = Bundle By Name(cluster=w553, "Wavelength, nm"=w554, "W-Sweep State"=Measurement.WavelengthSweeping.State--Enum."Wait for Wavelength set", "Next Step"="Measurement: OPA >> Set Shutter state Open\nMeasurement: Pause >>  Integration time") -> (w552:T22)
            n203 = call <vilib>:"Add State(s) to Queue__jki_lib_state_machine.vi"("State(s) in Front (\"\")"="Measurement: SMU >> Set Voltage\nMeasurement: SMU >> Set Output Enable", "State(s) in (\"\")"="Measurement: OPA >> Set Wavelength") -> ("States Out"=w549:string)  [unwired: 13 in]
            n204 = call <vilib>:"Add State(s) to Queue__jki_lib_state_machine.vi"("State(s) in Front (\"\")"=w549, "State(s) in (\"\")"=w558) -> ("States Out"=w557:string)  [unwired: 13 in]
          }
          frame "Macro: Measurement Stop" {
            n205 = Unbundle By Name(w563) -> ("Self Reference"=w562:refnum<class "Measurement.WavelengthSweeping.lvclass">)
            n206 = call "Measurement.OnFinished.vi"("error in (no error)"=w561, "Finished"=T7 TRUE, "Measurement in"=w562) -> ("error out"=w560:errorcluster)  [unwired: 7 in, 1 out]
            n207 = Bundle By Name(cluster=w563, "W-Sweep State"=Measurement.WavelengthSweeping.State--Enum."Stoppped") -> (w564:T22)
            n208 = call <vilib>:"Add State(s) to Queue__jki_lib_state_machine.vi"("State(s) in Front (\"\")"="Measurement: SMU >> Set Output Disable", "State(s) in (\"\")"="Measurement: OPA >> Set Shutter state Close") -> ("States Out"=w566:string)  [unwired: 13 in]
            n209 = call <vilib>:"Add State(s) to Queue__jki_lib_state_machine.vi"("State(s) in Front (\"\")"=w566, "State(s) in (\"\")"=w571) -> ("States Out"=w570:string)  [unwired: 13 in]
          }
          frame "---------- Process ----------" {
            # "Template Separator\n(You can make a copy of, or modify, this frame)"
            n210 = call <vilib>:"Add State(s) to Queue__jki_lib_state_machine.vi"("State(s) in (\"\")"=w576) -> ("States Out"=w575:string)  [unwired: 14 in]
          }
          frame "Process: Sync" {
            n211 = Unbundle By Name(w584) -> ("Self Reference"=w580:refnum<class "Measurement.WavelengthSweeping.lvclass">)
            n212 = call <vilib>:"WaitOnProcessSync.vi"("error in (no error)"=w579, "SMO"=w580) -> ("error out"=w578:errorcluster, "Don't run?"=w583:bool)  [unwired: 7 in, 1 out]
            n213 = Select(t="Data: Cleanup\nEvents: Unregister\nExit", s=w583, f="") -> (s? t:f=w577:string)
            n214 = call <vilib>:"Add State(s) to Queue__jki_lib_state_machine.vi"("State(s) in Front (\"\")"=w577, "State(s) in (\"\")"=w587) -> ("States Out"=w586:string)  [unwired: 13 in]
          }
          frame "---------- Events ----------" {
            # "Template Separator\n(You can make a copy of, or modify, this frame)"
            n215 = call <vilib>:"Add State(s) to Queue__jki_lib_state_machine.vi"("State(s) in (\"\")"=w592) -> ("States Out"=w591:string)  [unwired: 14 in]
          }
          frame "Events: Register" {
            # "Static Dependencies\nPublic Events"
            # "Measurement base\nProtected events"
            # "Base Class Protected Events"
            n216 = Unbundle By Name(w596) -> ("Self Reference"=w609:refnum<class "Measurement.WavelengthSweeping.lvclass">)
            n217 = Unbundle By Name(w596) -> ("Dependencies.OPM"=w605:refnum<class "OPM.lvclass">)
            n218 = Unbundle By Name(w596) -> ("Dependencies.SMU"=w607:refnum<class "SMU.lvclass">)
            n219 = Unbundle By Name(w596) -> ("Dependencies.OPA"=w595:refnum<class "OPA.lvclass">)
            n220 = Unbundle By Name(w596) -> ("Dependencies.LIA"=w606:refnum<class "LIA.lvclass">)
            n221 = call "Measurement.GetProtectedEventsRegistration.vi"("Measurement in"=w609) -> ("error out"=w601:errorcluster, "Measurement Protected Events"=w608:refnum<event-registration>)  [unwired: 8 in, 1 out]
            n222 = call <vilib>:"GetProtectedEvents.vi"("SMO"=w609) -> ("error out"=w613:errorcluster, "SMO Protected Events"=w615:T26)  [unwired: 8 in, 1 out]
            n223 = call "SMU.GetPublicEventsRegistration.vi"("SMU"=w607) -> ("error out"=w600:errorcluster, "SMU Public Events"=w604:refnum<event-registration>)  [unwired: 8 in, 1 out]
            n224 = call "LIA.GetPublicEventsRegistration.vi"("LIA"=w606) -> ("error out"=w599:errorcluster, "LIA Public Events"=w603:refnum<event-registration>)  [unwired: 8 in, 1 out]
            n225 = call "OPM.GetPublicEventsRegistration.vi"("PM"=w605) -> ("error out"=w598:errorcluster, "OPM Public Events"=w602:refnum<event-registration>)  [unwired: 8 in, 1 out]
            n226 = call "OPA.GetPublicEventsRegistration.vi"("OPA"=w595) -> ("error out"=w593:errorcluster, "OPA Public Events"=w594:refnum<event-registration>)  [unwired: 8 in, 1 out]
            n227 = register-events(w615) -> (reference out=w610:refnum<event-registration>, error out=w614:errorcluster)  [unwired: 2 in]
            n228 = Bundle("Event Registration Refnum"=w610, "Measurement Protected Events"=w608, "SMU Public Events"=w604, "LIA Public Events"=w603, "OPM Public Events"=w602, "OPA Public Events"=w594) -> (w611:T27)  [unwired: 1 in]
            n229 = Merge Errors(w614, w613, w601, w600, w599, w598, w593, w597) -> (w612:errorcluster)
            n230 = call <vilib>:"Add State(s) to Queue__jki_lib_state_machine.vi"("State(s) in (\"\")"=w617) -> ("States Out"=w616:string)  [unwired: 14 in]
          }
          frame "Events: Unregister" {
            n231 = Unregister For Events(event registration refnum=w620, error in=w619) -> (error out=w618:errorcluster)
            n232 = call <vilib>:"Clear Errors.vi"("error in (no error)"=w618) -> ()  [unwired: 5 in, 2 out]
            n233 = call <vilib>:"Add State(s) to Queue__jki_lib_state_machine.vi"("State(s) in (\"\")"=w623) -> ("States Out"=w622:string)  [unwired: 14 in]
          }
          frame "---------- API ----------" {
            n234 = call <vilib>:"Add State(s) to Queue__jki_lib_state_machine.vi"("State(s) in (\"\")"=w628) -> ("States Out"=w627:string)  [unwired: 14 in]
          }
          frame "Action: Initialize" {
            n235 = call-dynamic "Measurement.Init.vi"("error in (no error)"=w637, "Measurement.WavelengthSweeping in"=w638) -> ("error out"=w636:errorcluster, "Result"=w631:bool, "Measurement.WavelengthSweeping out"=w635:refnum<class "Measurement.WavelengthSweeping.lvclass">)  [unwired: 6 in, 1 out]
            n236 = case shown="False" w631 {
              tunnel: w636 -> [w645 w648]
              tunnel: [w644 w648] -> w634
              frame False {
                n237 = call <vilib>:"Error Cluster From Error Code.vi"("error in (no error)"=w645, "error message (\"\")"="Measurement Initialization failure" ("source"), "error code (0)"=-8000 ("code")) -> ("error out"=w644:errorcluster)  [unwired: 6 in]
              }
              frame True {
              }
            }
            n238 = call "Measurement.OnInitialized.vi"("error in (no error)"=w634, "Initialized"=w631, "Measurement in"=w635) -> ("error out"=w629:errorcluster)  [unwired: 7 in, 1 out]
            n239 = case shown="True" w631 {
              tunnel: [Measurement.State--Enum."Uninitialized" ("State") Measurement.State--Enum."Initialized" ("State")] -> w630
              frame False {
              }
              frame True {
              }
            }
            n240 = Bundle By Name(cluster=w633, "Meas State"=w630, "Initialized"=w631) -> (w632:T22)
            n241 = call <vilib>:"Add State(s) to Queue__jki_lib_state_machine.vi"("State(s) in (\"\")"=w641) -> ("States Out"=w640:string)  [unwired: 14 in]
          }
          frame "Action: Uninitialize" {
            n242 = call-dynamic "Measurement.Uninit.vi"("error in (no error)"=w657, "Measurement.WavelengthSweeping in"=w658) -> ("error out"=w655:errorcluster, "Measurement.WavelengthSweeping out"=w656:refnum<class "Measurement.WavelengthSweeping.lvclass">)  [unwired: 8 in]
            n243 = call "Measurement.OnUninitialized.vi"("error in (no error)"=w655, "Uninitialized (True)"=T8 TRUE ("Uninitialized"), "Measurement in"=w656) -> ("error out"=w654:errorcluster)  [unwired: 7 in, 1 out]
            n244 = Bundle By Name(cluster=w652, "Initialized"=FALSE, "Meas State"=Measurement.State--Enum."Uninitialized" ("State")) -> (w651:T22)
            n245 = call <vilib>:"Add State(s) to Queue__jki_lib_state_machine.vi"("State(s) in (\"\")"=w661) -> ("States Out"=w660:string)  [unwired: 14 in]
          }
        }
      }
    }
    frame Error {
    }
  }
  n246 = call-parent "Process.vi"("error in"=w8, "SMO"=w7) -> ("error out"=w5:errorcluster, "SMO out"=→"Measurement.WavelengthSweeping out":refnum<class "Measurement.WavelengthSweeping.lvclass">)  [unwired: 8 in]
  n247 = Merge Errors(w5, w4) -> (→"error out":errorcluster)
